vi "Manip1.vi"() -> ()   [LabVIEW 2021]
panel:
  in  "A":dbl
  out "C":dbl
  in  "B":dbl
  in  "y":dbl
  in  "x":dbl
  out "x+y":dbl
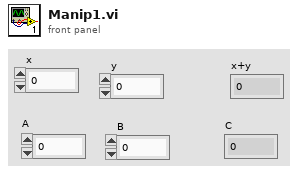
[diagram p1: front panel]
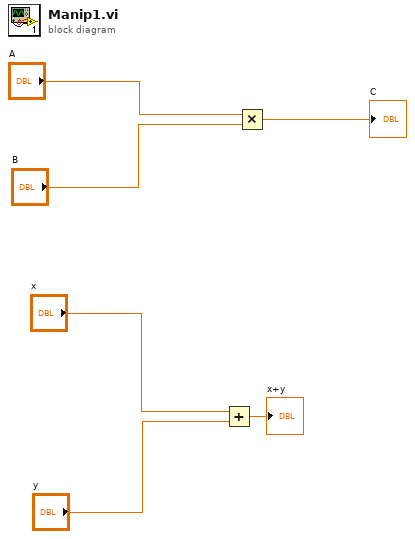
[diagram p0: block diagram]
diagram:
  n1 = Add(x="x", y="y") -> (x+y=→"x+y":dbl)
  n2 = Multiply(x="A", y="B") -> (x*y=→"C":dbl)
